vi "interpolate - with calibration array.vi"(1 "Input Number":dbl) -> (0 "Interpolated Function Value":dbl)   [LabVIEW 2009, in "Varian Magnet.lvclass"]
doc: "Instructions: Open up this VI and enter in the appropriate calibration array (x-values in left-hand column, y-values in right-hand column). Drag the array downward if needed. When done entering in the calibration, right click the array, and click \"Data Operations -> Make Current Value Default\". Then re-save the file.\n\nTo use: Give the function an input number. It will figure out the interpolated function value."
uses:
  Varian Magnet.lvclass
  <vilib>/gmath/NI_Gmath.lvlib
panel:
  in  "Calibration Array":dbl[][](array[numeric])=[[0.02028168565397942, 4.745924262319057, 0.0, 0.0], [0.03017065128325186, 4.5319418461993575, 0.0, 0.0], [0.04008593588171383, 4.291747225086936, 0.0, 0.0], [0.04961340272829584, 4.055797682959657, 0.0, 0.0], [0.060007847383471646, 3.9893767679833863, 0.0, 0.0], [0.06986089536067375, 3.8435858681045865, 0.0, 0.0], [0.07964876518476555, 3.7216828229593566, 0.0, 0.0], [0.08978218759256834, 3.621000454693889, 0.0, 0.0], [0.09976419851879875, 3.5332108262984887, 0.0, 0.0], [0.10998849877903805, 3.4373168617617607, 0.0, 0.0], [0.11946967520333979, 3.3044746120704795, 0.0, 0.0], [0.12961145775429678, 3.249818450445633, 0.0, 0.0], [0.13994908439951653, 3.1821531851333638, 0.0, 0.0], [0.1500442668932616, 3.097089044299053, 0.0, 0.0], [0.1600383535818261, 3.0498883525690736, 0.0, 0.0], [0.17031467251058097, 3.0029186007401782, 0.0, 0.0], [0.18011167656515614, 2.8846972313747887, 0.0, 0.0], [0.1898088233542773, 2.7888478327337713, 0.0, 0.0], [0.19981359244798336, 2.721364364818148, 0.0, 0.0], [0.2099138839181005, 2.6401910283790757, 0.0, 0.0], [0.22013121739237784, 2.590112147385445, 0.0, 0.0], [0.2302781089197069, 2.56922390998729, 0.0, 0.0], [0.23997138527218254, 2.457172705714308, 0.0, 0.0], [0.2494914208804052, 2.3604966753422576, 0.0, 0.0], [0.2601835795223535, 2.349912182261242, 0.0, 0.0], [0.27003894976154286, 2.267044644830819, 0.0, 0.0], [0.28001182645728995, 2.201328114354037, 0.0, 0.0], [0.29020717585142086, 2.129140576588889, 0.0, 0.0], [0.2999970583025683, 2.081906648521364, 0.0, 0.0], [0.3100600387634228, 2.0044119886624556, 0.0, 0.0], [0.3199596867978368, 1.9357566715210517, 0.0, 0.0], [0.32941903395945804, 1.851804862486773, 0.0, 0.0], [0.33989413851432615, 1.8052344993904144, 0.0, 0.0], [0.34985184309842277, 1.7509343498758034, 0.0, 0.0], [0.3600767626285253, 1.7213623482590878, 0.0, 0.0], [0.369382221229121, 1.608820744129774, 0.0, 0.0], [0.38043015040752426, 1.6058012456762079, 0.0, 0.0], [0.38971594718996083, 1.470102028888871, 0.0, 0.0], [0.39981948982686033, 1.421614428539224, 0.0, 0.0], [0.4104091593064355, 1.3886687637686794, 0.0, 0.0], [0.4197714359169873, 1.3042291208211823, 0.0, 0.0], [0.42995130356453604, 1.2665389516316452, 0.0, 0.0], [0.44026415941522457, 1.2070880446776138, 0.0, 0.0], [0.4499839095543553, 1.1135840022948118, 0.0, 0.0], [0.45952747741738276, 1.0180900630185559, 0.0, 0.0], [0.4698932808413817, 1.003058169426728, 0.0, 0.0], [0.4795065165640282, 0.9098165020754078, 0.0, 0.0], [0.48989306552844714, 0.9064234311520589, 0.0, 0.0], [0.5002949414219823, 0.8604237645682591, 0.0, 0.0], [0.50996406624979, 0.7854789728451561, 0.0, 0.0], [0.5193074551295117, 0.6745734255709245, 0.0, 0.0], [0.5296974100781786, 0.6339896533848023, 0.0, 0.0], [0.5404048956492431, 0.6136023494421956, 0.0, 0.0], [0.5503056274059178, 0.5682706426287631, 0.0, 0.0], [0.5600482905299902, 0.4948276872357007, 0.0, 0.0], [0.569926573754121, 0.4255113563969392, 0.0, 0.0], [0.5798183260977783, 0.338844470666983, 0.0, 0.0], [0.589730204711992, 0.28414051558182396, 0.0, 0.0], [0.6002221843706347, 0.2673066488308337, 0.0, 0.0], [0.6100777094272899, 0.219752461421066, 0.0, 0.0], [0.6201456440470506, 0.1307111267288926, 0.0, 0.0], [0.6301878789674853, 0.09635066669746253, 0.0, 0.0], [0.6395294100376171, -0.009997293550217862, 0.0, 0.0], [0.6500552947212743, -0.024512842600641654, 0.0, 0.0], [0.6601065090547265, -0.07278964300877125, 0.0, 0.0], [0.6698891150849804, -0.14253020632150612, 0.0, 0.0], [0.6803826429182812, -0.16848065164434653, 0.0, 0.0], [0.6899725012035887, -0.2678505790794944, 0.0, 0.0], [0.6999085313424707, -0.3208655200427105, 0.0, 0.0], [0.7101747871359472, -0.37206074816062473, 0.0, 0.0], [0.7204003259359129, -0.42917018537576546, 0.0, 0.0], [0.729864162804043, -0.5061421963986503, 0.0, 0.0], [0.7401647880749316, -0.5256122440128862, 0.0, 0.0], [0.7499038903972899, -0.6098927323173143, 0.0, 0.0], [0.7598855916885889, -0.6613207820219337, 0.0, 0.0], [0.7699823223569922, -0.7532722413887796, 0.0, 0.0], [0.7798873890027098, -0.7897911206259668, 0.0, 0.0], [0.7903592423907957, -0.8069822513016809, 0.0, 0.0], [0.0, 0.0, 0.1, 3.66], [0.0, 0.0, 0.2, 2.852], [0.0, 0.0, 0.3, 2.213], [0.0, 0.0, 0.4, 1.55], [0.0, 0.0, 0.5, 0.965], [0.0, 0.0, 0.6, 0.408], [0.0, 0.0, 0.7, -0.165], [0.0, 0.0, 0.8, -0.738]]
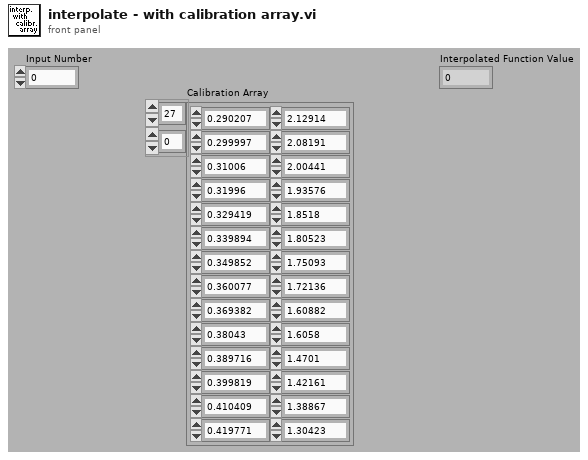
[diagram p1: front panel]
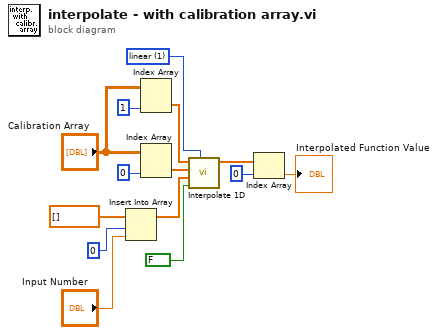
[diagram p0: block diagram]
diagram:
  w9 = 1 items=["nearest", "linear", "spline", "cubic Hermite", "Lagrange"] ("method")
  n1 = Insert Into Array(array=dbl[] [], index=0, new element="Input Number") -> (w4:dbl[])
  n2 = Index Array(array="Calibration Array", index (col)=1 ("disabled index (col)")) -> (element=w10:dbl[])  [unwired: 1 in]
  n3 = Index Array(array="Calibration Array", index (col)=0 ("disabled index (col)")) -> (element=w13:dbl[])  [unwired: 1 in]
  n4 = call <vilib>:"Interpolate 1D.vi"("method"=w9, "X is monotonic"=FALSE, "xi"=w4, "X"=w13, "Y"=w10) -> ("yi"=w2:dbl[])  [unwired: 1 in, 5 out]
  n5 = Index Array(array=w2, index=0) -> (element=→"Interpolated Function Value":dbl)
